vi "Combined_VIs.vi"() -> ()   [LabVIEW 2017]
uses:
  <vilib>/Plasmionique/MB Master/MB_Master_TCP/MB_Master_TCP.lvclass
  <vilib>/Plasmionique/MB Master/MB Master.lvlib
  ff2c3a55-e4d3-403f-981d-a63d6485aa43.vi
  <vilib>/Plasmionique/MB Master/MB_Master_Serial/MB_Master_Serial.lvclass
  C:/Program Files (x86)/National Instruments/LabVIEW 2017/vi.lib/Plasmionique/MB Master/MB_Master/MB_Master.lvclass
panel:
  in  "Serial Config":cluster{"baud rate (bps)":u32, "stop bits":u16}
  in  "Slave ID":u8=1
  in  "VISA Resource":refnum<visa-resource-name>
  out "Binary Conversion":i16
  out "Inverter Error?":string="Inverter not ready!"
  out "Heartbeat Value to BMS":u16
  out "Battery Idle?":string="Battery is Idle"
  out "BMS Error?":string="Critical Fault Occurred!\nContact Primus\nPower Service!"
  out "BMS IP Address":string
  out "Inverter IP Address":string
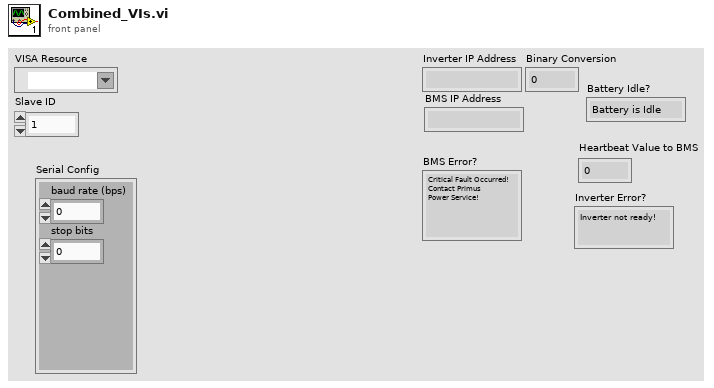
[diagram p1: front panel]
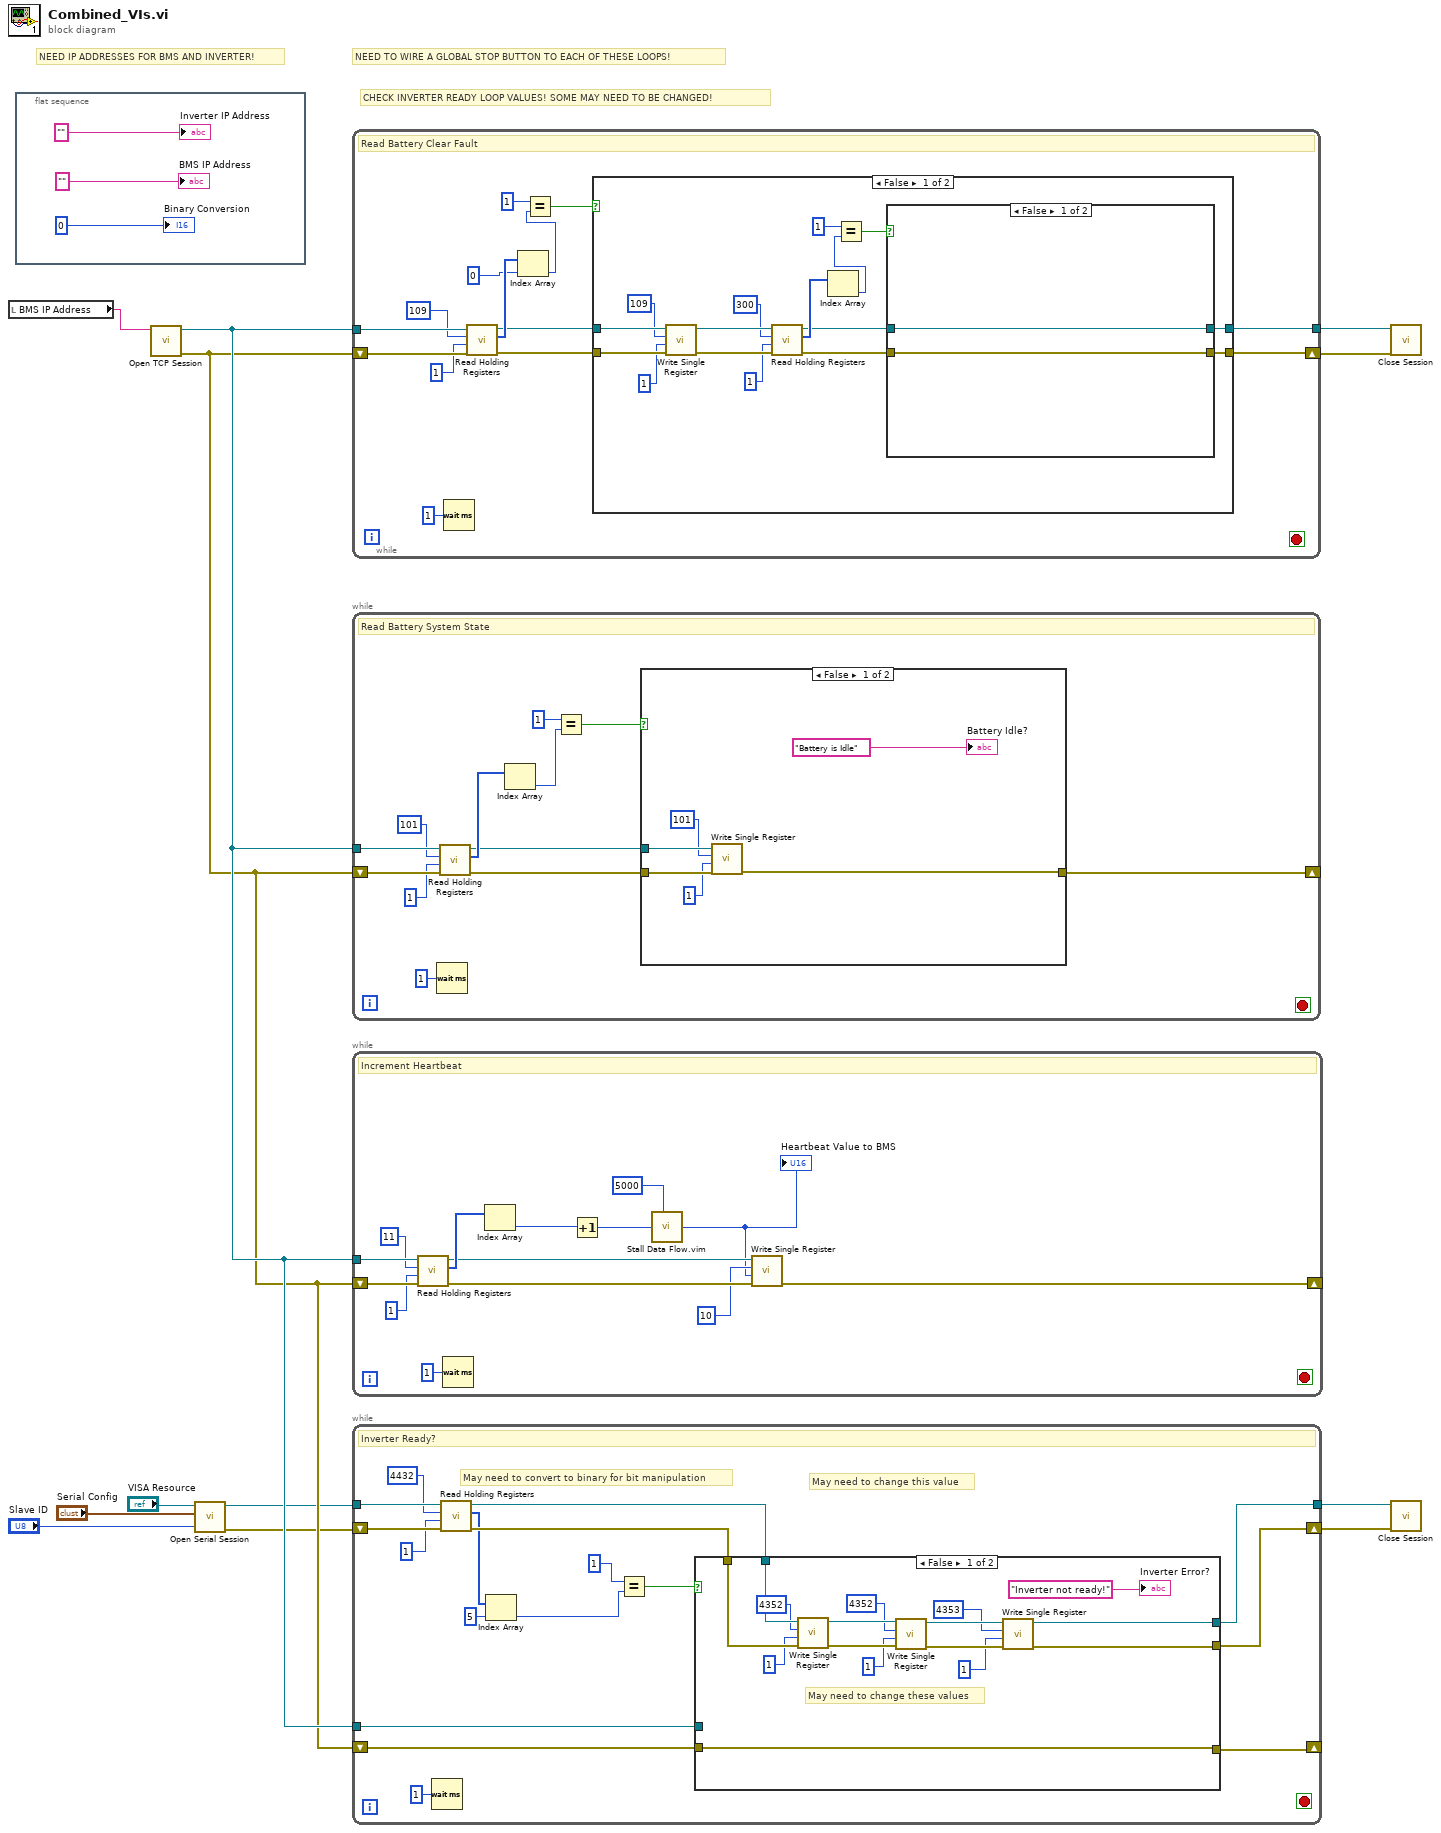
[diagram p0: block diagram]
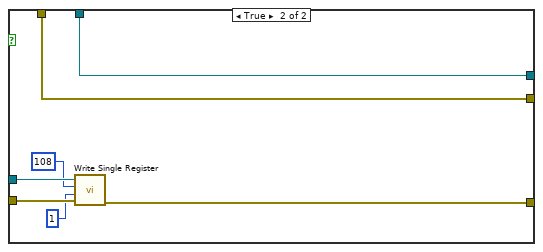
[diagram p2: hidden frame]
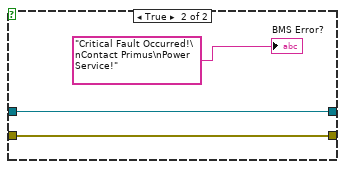
[diagram p4: hidden frame]
diagram:
  # "NEED IP ADDRESSES FOR BMS AND INVERTER!"
  # "CHECK INVERTER READY LOOP VALUES! SOME MAY NEED TO BE CHANGED!"
  # "NEED TO WIRE A GLOBAL STOP BUTTON TO EACH OF THESE LOOPS!"
  n1 = local read "BMS IP Address"() -> (w12:string)
  n2 = flat-sequence {
    frame #0 {
      "Inverter IP Address" <- ""
      "BMS IP Address" <- ""
      "Binary Conversion" <- 0
    }
  }
  n3 = call <vilib>:"Open TCP Session.vi"("IP Address"=w12) -> ("error out"=w8:errorcluster, "MB_TCP session"=w9:refnum<class "MB_Master_TCP.lvclass">)  [unwired: 9 in]
  n4 = call <vilib>:"Open Serial Session.vi"("Slave ID"="Slave ID", "Serial Config"="Serial Config", "VISA Resource"="VISA Resource") -> ("Error out"=w1:errorcluster, "MB_Serial session"=w2:refnum<class "MB_Master_Serial.lvclass">)  [unwired: 7 in]
  n5 = while {
    tunnel: w9 -> [w29]
    shift-right: [w17] -> w10
    shift-left: w8 -> [w28]
    tunnel: [w16] -> w11
    stop <- _ stop-if-true
    # "Read Battery Clear Fault"
    n6 = Wait (ms)(milliseconds to wait=u32 1) -> ()  [unwired: 1 out]
    n7 = call <vilib>:"Read Holding Registers.vi"("error in (no error)"=w28, "quantity"=u16 1, "starting address"=u16 109, "MB session in"=w29) -> ("error out"=w18:errorcluster, "Registers"=w25:u16[], "MB session out"=w19:refnum<class "MB_Master_TCP.lvclass">)  [unwired: 5 in]
    n8 = Index Array(array=w25, index=0) -> (element=w23:u16)
    n9 = Equal?(x=u16 1, y=w23) -> (x = y?=w20:bool)
    n10 = case shown="False" w20 {
      tunnel: w19 -> [w45 w52]
      tunnel: w18 -> [w44 w51]
      tunnel: [w31 w52] -> w16
      tunnel: [w30 w51] -> w17
      frame False {
        n11 = call <vilib>:"Write Single Register.vi"("error in (no error)"=w44, "value"=u16 1, "address"=u16 109, "MB session in"=w45) -> ("error out"=w40:errorcluster, "MB session out"=w41:refnum<class "MB_Master_TCP.lvclass">)  [unwired: 6 in]
        n12 = call <vilib>:"Read Holding Registers.vi"("error in (no error)"=w40, "quantity"=u16 1, "starting address"=u16 300, "MB session in"=w41) -> ("error out"=w32:errorcluster, "Registers"=w37:u16[], "MB session out"=w33:refnum<class "MB_Master_TCP.lvclass">)  [unwired: 5 in]
        n13 = Index Array(array=w37) -> (element=w36:u16)  [unwired: 1 in]
        n14 = Equal?(x=u16 1, y=w36) -> (x = y?=w34:bool)
        n15 = case shown="False" w34 {
          tunnel: w33 -> [w47 w50]
          tunnel: w32 -> [w46 w49]
          tunnel: [w47 w50] -> w31
          tunnel: [w46 w49] -> w30
          frame False {
          }
          frame True {
            "BMS Error?" <- "Critical Fault Occurred!\nContact Primus\nPower Service!"
          }
        }
      }
      frame True {
      }
    }
  }
  n16 = while {
    tunnel: w9 -> [w64]
    shift-right: [w53] -> _
    shift-left: w8 -> [w63]
    stop <- _ stop-if-true
    # "Read Battery System State"
    n17 = Wait (ms)(milliseconds to wait=u32 1) -> ()  [unwired: 1 out]
    n18 = call <vilib>:"Read Holding Registers.vi"("error in (no error)"=w63, "quantity"=u16 1, "starting address"=u16 101, "MB session in"=w64) -> ("error out"=w54:errorcluster, "Registers"=w60:u16[], "MB session out"=w55:refnum<class "MB_Master_TCP.lvclass">)  [unwired: 5 in]
    n19 = Index Array(array=w60) -> (element=w59:u16)  [unwired: 1 in]
    n20 = Equal?(x=u16 1, y=w59) -> (x = y?=w56:bool)
    n21 = case shown="False" w56 {
      tunnel: w55 -> [w70 _]
      tunnel: w54 -> [w69 w71]
      tunnel: [w66 w71] -> w53
      frame False {
        n22 = call <vilib>:"Write Single Register.vi"("error in (no error)"=w69, "value"=u16 1, "address"=u16 101, "MB session in"=w70) -> ("error out"=w66:errorcluster)  [unwired: 6 in, 1 out]
        "Battery Idle?" <- "Battery is Idle"
      }
      frame True {
      }
    }
  }
  n23 = while {
    tunnel: w9 -> [w84]
    shift-right: [w72] -> _
    shift-left: w8 -> [w83]
    stop <- _ stop-if-true
    # "Increment Heartbeat"
    n24 = call <vilib>:"Read Holding Registers.vi"("error in (no error)"=w83, "quantity"=u16 1, "starting address"=u16 11, "MB session in"=w84) -> ("error out"=w75:errorcluster, "Registers"=w80:u16[], "MB session out"=w76:refnum<class "MB_Master_TCP.lvclass">)  [unwired: 5 in]
    n25 = Wait (ms)(milliseconds to wait=u32 1) -> ()  [unwired: 1 out]
    n26 = Index Array(array=w80) -> (element=w79:u16)  [unwired: 1 in]
    n27 = Increment(x=w79) -> (x+1=w78:u16)
    n28 = call "Stall Data Flow.vim"("value in"=w78, "milliseconds to wait"=u32 5000) -> ("value out"=w73:u16)  [unwired: 1 out]
    "Heartbeat Value to BMS" <- w73
    n29 = call <vilib>:"Write Single Register.vi"("error in (no error)"=w75, "value"=w73, "address"=u16 10, "MB session in"=w76) -> ("error out"=w72:errorcluster)  [unwired: 6 in, 1 out]
  }
  n30 = while {
    tunnel: w2 -> [w102]
    tunnel: w9 -> [w97]
    shift-right: [w89] -> w6
    shift-left: w1 -> [w101]
    shift-right: [w91] -> _
    shift-left: w8 -> [w96]
    tunnel: [w90] -> w7
    stop <- _ stop-if-true
    # "May need to convert to binary for bit manipulation"
    # "May need to change this value"
    # "Inverter Ready?"
    n31 = Wait (ms)(milliseconds to wait=u32 1) -> ()  [unwired: 1 out]
    n32 = call <vilib>:"Read Holding Registers.vi"("error in (no error)"=w101, "quantity"=u16 1, "starting address"=u16 4432, "MB session in"=w102) -> ("error out"=w94:errorcluster, "Registers"=w88:u16[], "MB session out"=w95:refnum<class "MB_Master_Serial.lvclass">)  [unwired: 5 in]
    n33 = Index Array(array=w88, index=5) -> (element=w87:u16)
    n34 = Equal?(x=u16 1, y=w87) -> (x = y?=w92:bool)
    n35 = case shown="False" w92 {
      tunnel: w97 -> [_ w125]
      tunnel: w96 -> [w118 w124]
      tunnel: w95 -> [w110 w121]
      tunnel: w94 -> [w109 w120]
      tunnel: [w116 w121] -> w90
      tunnel: [w115 w120] -> w89
      tunnel: [w118 w119] -> w91
      frame False {
        # "May need to change these values"
        n36 = call <vilib>:"Write Single Register.vi"("error in (no error)"=w109, "value"=u16 1, "address"=u16 4352, "MB session in"=w110) -> ("error out"=w111:errorcluster, "MB session out"=w112:refnum<class "MB_Master_Serial.lvclass">)  [unwired: 6 in]
        n37 = call <vilib>:"Write Single Register.vi"("error in (no error)"=w111, "value"=u16 1, "address"=u16 4352, "MB session in"=w112) -> ("error out"=w114:errorcluster, "MB session out"=w113:refnum<class "MB_Master_Serial.lvclass">)  [unwired: 6 in]
        n38 = call <vilib>:"Write Single Register.vi"("error in (no error)"=w114, "value"=u16 1, "address"=u16 4353, "MB session in"=w113) -> ("error out"=w115:errorcluster, "MB session out"=w116:refnum<class "MB_Master_Serial.lvclass">)  [unwired: 6 in]
        "Inverter Error?" <- "Inverter not ready!"
      }
      frame True {
        n39 = call <vilib>:"Write Single Register.vi"("error in (no error)"=w124, "value"=u16 1, "address"=u16 108, "MB session in"=w125) -> ("error out"=w119:errorcluster)  [unwired: 6 in, 1 out]
      }
    }
  }
  n40 = call-dynamic "Close Session.vi"("error in (no error)"=w10, "MB TCP session"=w11) -> ()  [unwired: 9 in, 1 out]
  n41 = call-dynamic "Close Session.vi"("error in (no error)"=w6, "MB_Serial session"=w7) -> ()  [unwired: 9 in, 1 out]
